vi "AddWeightedImagesARGB.vi"(5 "B":dbl=0.5, 6 "C (Default: 0)":dbl, 7 "A":dbl=0.5, 8 "error in (no error)":errorcluster, 9 "ARGB Image Destination":refnum<data-value>, 10 "ARGB Image B":refnum<data-value>, 11 "ARGB Image A":refnum<data-value>) -> (0 "error out":errorcluster, 3 "ARGB Image Destination (duplicate)":refnum<data-value>)   [LabVIEW 2020, in "g_ar_toolkit.image.lvlib"]
uses:
  g_ar_toolkit.image.lvlib
  <vilib>/Utility/error.llb/Error Cluster From Error Code.vi
  000615f7-9334-4574-8f7b-324cbbba12df.vi
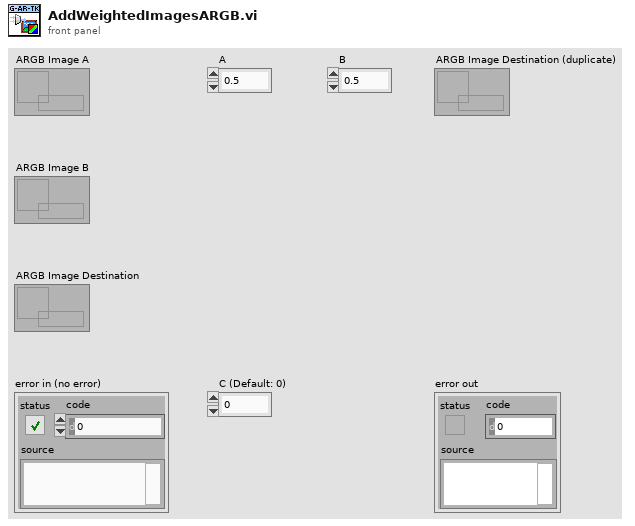
[diagram p1: front panel]
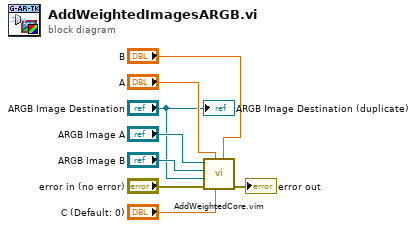
[diagram p0: block diagram]
diagram:
  n1 = call "AddWeightedCore.vim"(5:"B"="B", "C"="C (Default: 0)", 7:"A"="A", "error in (no error)"="error in (no error)", "Dst"="ARGB Image Destination", 10:"B"="ARGB Image B", 11:"A"="ARGB Image A") -> ("error out"=→"error out":errorcluster)  [unwired: 4 in]
  "ARGB Image Destination (duplicate)" <- "ARGB Image Destination"
